vi "AUTOFOCUS_read_QPD_signal_calibration.vi"(4 "previous count":u32, 5 "iteration":i32, 6 "error in":errorcluster, 7 "z":dbl, 8 "channel":bool) -> (0 "error out":errorcluster, 1 "new count":u32, 2 "QPD":dbl, 3 "Calibration":cluster{"Y":dbl[], "Y":dbl[]}[](graph))   [LabVIEW 2015]
uses:
  GLOBAL/Global_FPGA.vi
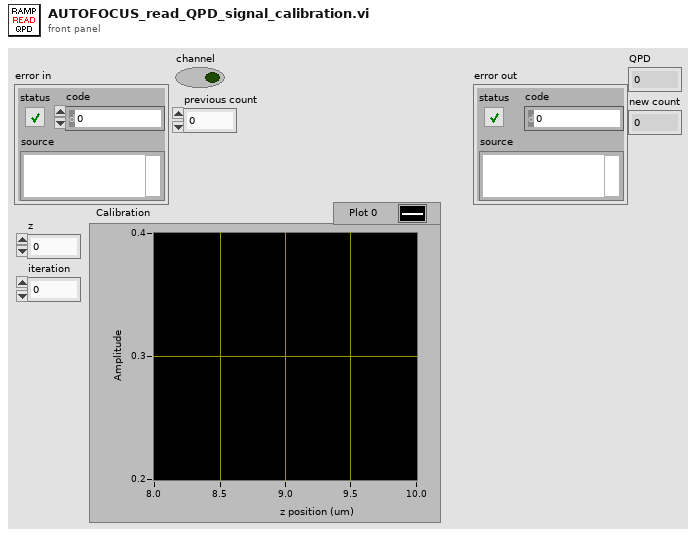
[diagram p1: front panel]
types:
  T1 = cluster{"X":sgl, "Y":sgl, "SUM":sgl, "count":u32}
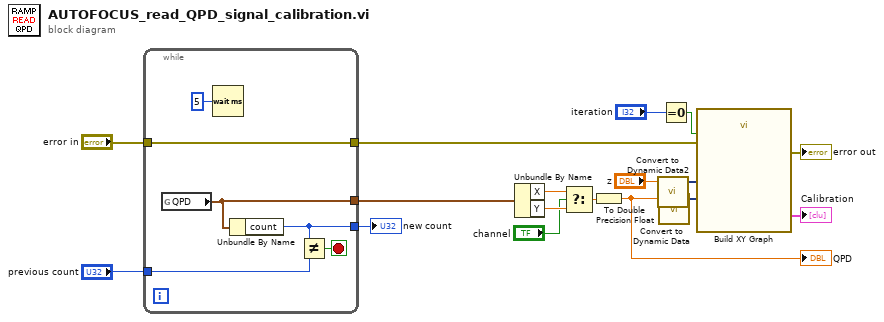
[diagram p0: block diagram]
diagram:
  n1 = while {
    tunnel: [w21] -> w13
    tunnel: "error in" -> [w23]
    tunnel: [w23] -> w4
    tunnel: "previous count" -> [w19]
    tunnel: [w18] -> w2
    stop <- w20 stop-if-true
    n2 = global read "Global_FPGA.vi" "QPD"() -> (w21:T1)
    n3 = Wait (ms)(milliseconds to wait=u32 5) -> ()  [unwired: 1 out]
    n4 = Unbundle By Name(w21) -> ("count"=w18:u32)
    n5 = Not Equal?(x=w18, y=w19) -> (x != y?=w20:bool)
  }
  "new count" <- w2
  n6 = Unbundle By Name(w13) -> ("X"=w12:sgl, "Y"=w11:sgl)
  n7 = Select(t=w12, s="channel", f=w11) -> (s? t:f=w8:sgl)
  n8 = To Double Precision Float(number=w8) -> (double precision float=w1:dbl)
  "QPD" <- w1
  n9 = call "Convert to Dynamic Data2"("Double"="z") -> ("Dynamic Data Type"=w16:dynamicdata)  [unwired: 3 in]
  n10 = call "Convert to Dynamic Data"("Double"=w1) -> ("Dynamic Data Type"=w15:dynamicdata)  [unwired: 3 in]
  n11 = Equal To 0?(x="iteration") -> (x = 0?=w14:bool)
  n12 = call "Build XY Graph"("error in (no error)"=w4, "Reset"=w14, "Y Input"=w15, "X Input"=w16) -> ("error out"=→"error out":errorcluster, "XY Graph"=→"Calibration":cluster{"X":dbl[], "Y":dbl[]}[])  [unwired: 6 in]
